vi "AdvanceRampProg.vi"(8 "error in (no error)":errorcluster, 11 "RampProgramModel in":refnum<class "RampProgramModel.lvclass">) -> (0 "error out":errorcluster, 2 "EndOfPrograms":bool, 3 "RampProgramModel out":refnum<class "RampProgramModel.lvclass">)   [LabVIEW 2013, in "RampProgramModel.lvclass"]
uses:
  RampProgramModel.lvclass
  RampProgramModel.lvclass/RampProgramModel.ctl
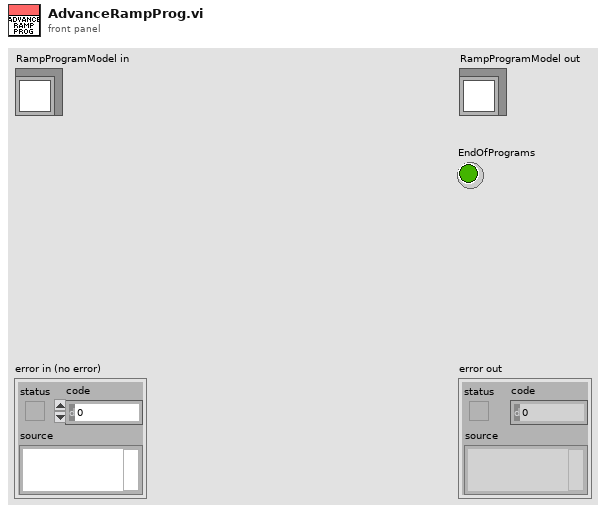
[diagram p1: front panel]
types:
  T1 = cluster{"SP (°C)":dbl, "Cooling rate (°C/min)":dbl, "Dwell Time @ SP (sec)":u32}[]
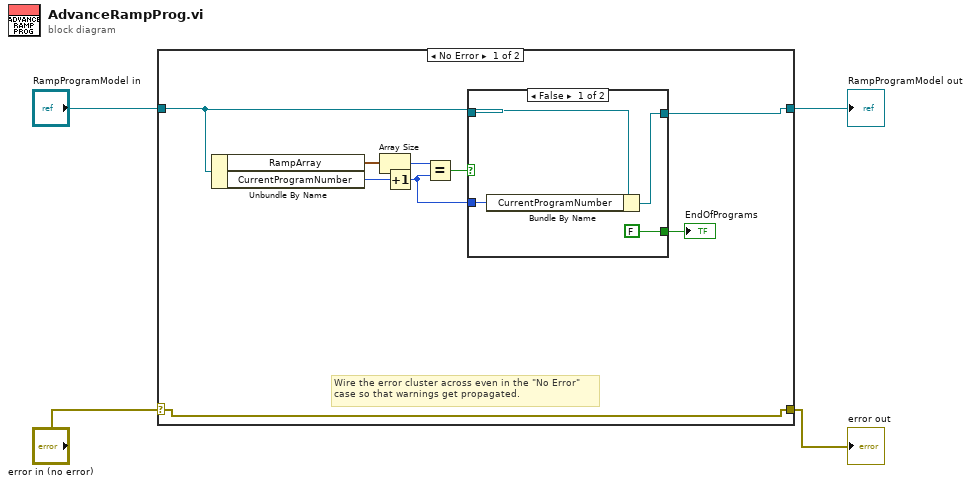
[diagram p0: block diagram]
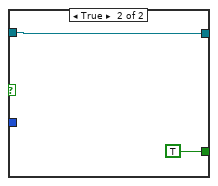
[diagram p2: hidden frame]
diagram:
  n1 = case shown="No Error" "error in (no error)" {
    selector: "error in (no error)" -> [w13 w21]
    tunnel: [w13 w21] -> w3
    tunnel: [w6 w20] -> w1
    tunnel: "RampProgramModel in" -> [w7 w20]
    frame No Error {
      # "Wire the error cluster across even in the \"No Error\"\ncase so that warnings get propagated."
      n2 = Unbundle By Name(w7) -> ("RampArray"=w12:T1, "CurrentProgramNumber"=w11:u32)
      n3 = Array Size(array=w12) -> (size(s)=w10:i32)
      n4 = Increment(x=w11) -> (x+1=w5:u32)
      n5 = Equal?(x=w10, y=w5) -> (x = y?=w9:bool)
      n6 = case shown="False" w9 {
        tunnel: [FALSE ("EndOfPrograms") TRUE ("EndOfPrograms")] -> w8
        tunnel: w7 -> [w16 w18]
        tunnel: [w15 w18] -> w6
        tunnel: w5 -> [w14 _]
        frame False {
          n7 = Bundle By Name(cluster=w16, "CurrentProgramNumber"=w14) -> (w15:refnum<class "RampProgramModel.lvclass">)
        }
        frame True {
        }
      }
      "EndOfPrograms" <- w8
    }
    frame Error {
    }
  }
  "error out" <- w3
  "RampProgramModel out" <- w1
